vi "aboutBenjaminR.vi"() -> ()   [LabVIEW 2017, in "shared.lvlib"]
doc: "About VI."
uses:
  <vilib>/Platform/browser.llb/Open URL in Default Browser (string).vi
  shared.lvlib
panel:
  out "Explore the project on GitHub":string
  # "BenjaminR's LabVIEW Extensions"
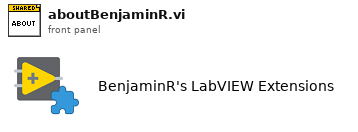
[diagram p1: front panel]
types:
  T1 = enum32{"Invalid", "Standard", "Closed", "Hidden", "Minimized", "Maximized"}
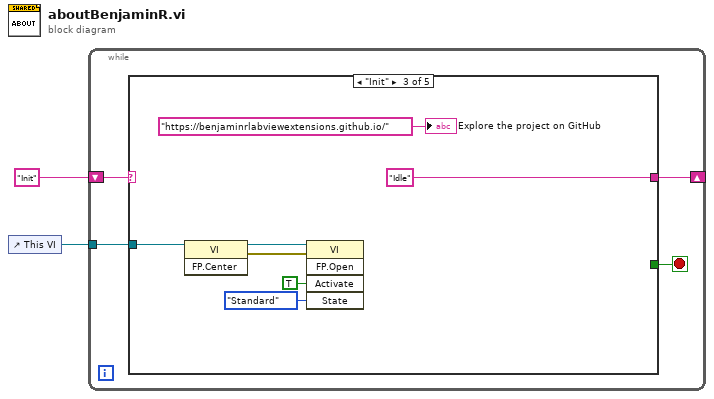
[diagram p0: block diagram]
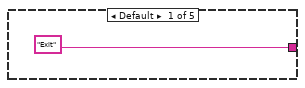
[diagram p2: hidden frame]
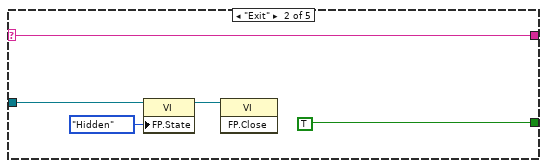
[diagram p3: hidden frame]
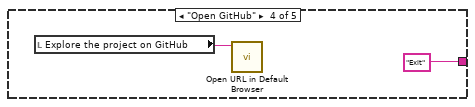
[diagram p4: hidden frame]
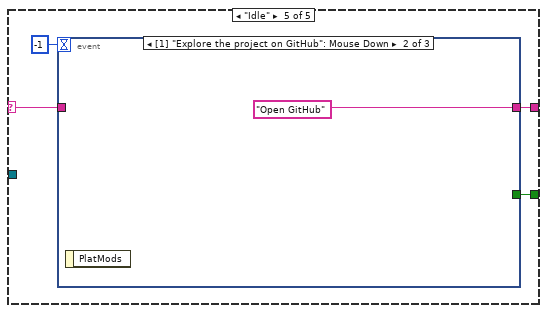
[diagram p5: hidden frame]
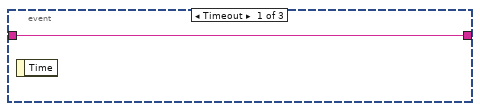
[diagram p6: hidden frame]
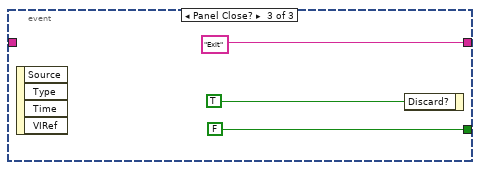
[diagram p7: hidden frame]
diagram:
  n1 = control-ref of="This VI"() -> (w1:refnum<vi>)
  n2 = while {
    shift-right: [w5] -> _
    shift-left: "Init" -> [w4]
    tunnel: w1 -> [w3]
    stop <- w6 stop-if-true
    n3 = case shown="\"Init\"" w4 {
      selector: w4 -> [_ w11 _ _ w22]
      tunnel: [_ TRUE _ _ w24] -> w6
      tunnel: ["Exit" w11 "Idle" "Exit" w23] -> w5
      tunnel: w3 -> [_ w10 w18 _ _]
      frame Default {
      }
      frame "Exit" {
        n4 = property class="VI"(reference=w10, "FP.State"=T1."Hidden" ("Front Panel Window:State")) -> (reference out=w9:refnum<vi>)  [unwired: 1 in, 1 out]
        n5 = invoke class="VI" method="FP.Close"(reference=w9) -> ()  [unwired: 2 in, 3 out]
      }
      frame "Init" {
        n6 = invoke class="VI" method="FP.Center"(reference=w18) -> (reference out=w17:refnum<vi>, error out=w14:errorcluster)  [unwired: 2 in, 1 out]
        n7 = invoke class="VI" method="FP.Open"(reference=w17, error in=w14, "Activate"=TRUE ("Activate?"), "State"=T1."Standard") -> ()  [unwired: 1 in, 5 out]
        "Explore the project on GitHub" <- "https://benjaminrlabviewextensions.github.io/" ("Explore the project on GitHub")
      }
      frame "Open GitHub" {
        n8 = local read "Explore the project on GitHub"() -> (w20:string)
        n9 = call-poly <vilib>:"Open URL in Default Browser.vi"("URL"=w20) -> ()  [unwired: 5 in, 2 out]
      }
      frame "Idle" {
        n10 = event shown="[1] \"Explore the project on GitHub\": Mouse Down" {
          selector: _ -> [_ _ _]
          dyn-events: _ -> [_ _ _]
          timeout: -1 -> [_ _ _]
          tunnel: [_ _ FALSE ("Discard?")] -> w24
          tunnel: w22 -> [w26 _ _]
          tunnel: [w26 "Open GitHub" "Exit"] -> w23
          event Timeout {
            n11 = event-data() -> ()  [unwired: 1 in, 1 out]
          }
          event "Explore the project on GitHub": Mouse Down {
            n12 = event-data() -> ()  [unwired: 1 in, 1 out]
          }
          event Panel Close? {
            n13 = event-data() -> ()  [unwired: 1 in, 4 out]
            n14 = event-data("Discard?"=TRUE) -> ()  [unwired: 1 in, 1 out]
          }
        }
      }
    }
  }
